vi "PM100D_Plot_ph.vi"(1 "Beam Name":string="Green Unshifted") -> ()   [LabVIEW 2012]
doc: "This VI shows how to communicate with a PM100D optical power/energy meter with SCPI commands.\n- Initializing the instrument\n- Getting system info\n- Setting parameters\n- Measurement configuration\n- Measuring queue\n- Fetching and displaying a measurement value\n- Closing the application"
panel:
  in  "Publish As Adam Channel":bool
  out "Wavelength nm":string="488"
  out "Waveform Chart":dbl(graph)
  out "Readout value":dbl format="%^#_9e"
  out "IDN String":string
  out "Sensor SN":string
  out "Sensor Name":string
  out "Sensor Flags":bool[](array[boolean])
  out "New":bool
  in  "Timeout [ms]":i32=1000
  in  "stop":bool
  in  "Readout Config":string(combo)="POW"
  out "Readout string":string
  out "Error log":string
  in  "Averaging Rate":i32=300
  # "1 Power Sensor"
  # "2 Energy Sensor"
  # "4"
  # "8"
  # "16 Response settable"
  # "32 Wavelength settable"
  # "64 Tau (time constant) settable"
  # "128"
  # "256 With temperature sensor"
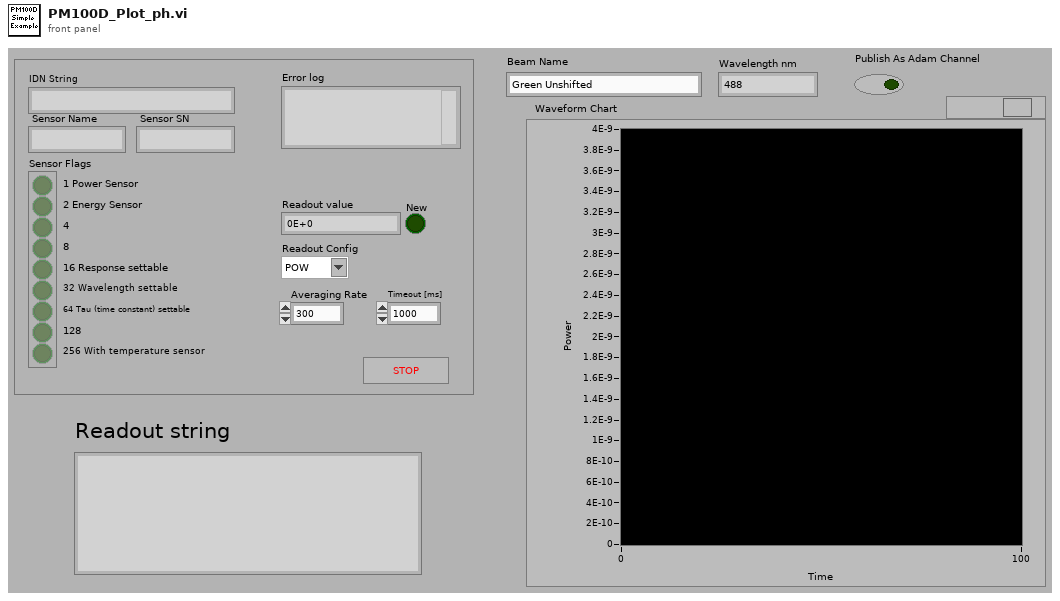
[diagram p1: front panel]
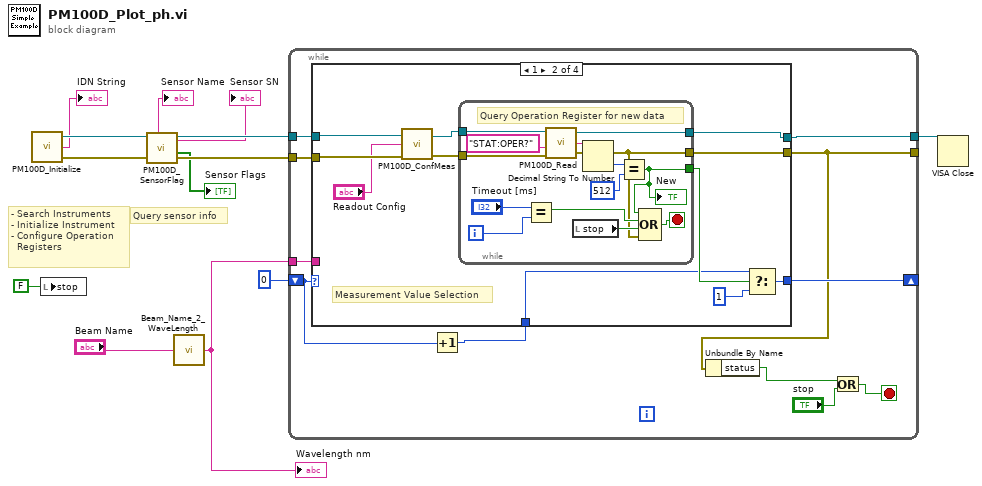
[diagram p0: block diagram]
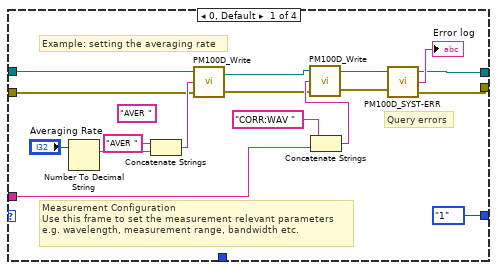
[diagram p2: hidden frame]
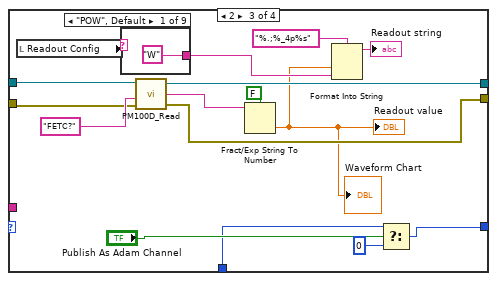
[diagram p3: hidden frame]
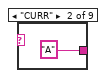
[diagram p4: hidden frame]
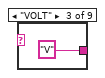
[diagram p5: hidden frame]
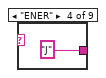
[diagram p6: hidden frame]
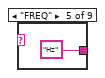
[diagram p7: hidden frame]
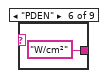
[diagram p8: hidden frame]
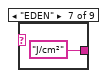
[diagram p9: hidden frame]
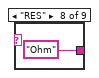
[diagram p10: hidden frame]
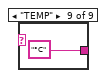
[diagram p11: hidden frame]
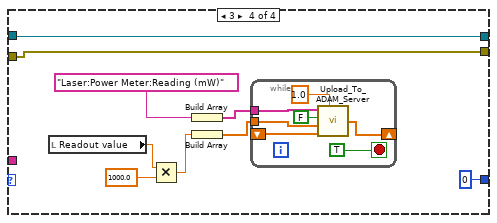
[diagram p12: hidden frame]
diagram:
  # "- Search Instruments\n- Initialize Instrument\n- Configure Operation\n  Registers"
  # "Query sensor info"
  n1 = call "PM100D_Initialize.vi"() -> ("error out"=w12:errorcluster, "Instrument"=→"IDN String":string, "VISA out"=w13:refnum<visa-resource-name>)  [unwired: 3 out]
  n2 = local write "stop"(FALSE ("stop")) -> ()
  n3 = call "PM100D_SensorFlag.vi"("error in (no error)"=w12, "VISA in"=w13) -> ("error out"=w10:errorcluster, "flags"=→"Sensor Flags":bool[], "VISA out"=w11:refnum<visa-resource-name>, "sn"=→"Sensor SN":string, "name"=→"Sensor Name":string)  [unwired: 5 out]
  n4 = call "Beam_Name_2_WaveLength.vi"("Beam Name"="Beam Name") -> ("Wavelength nm"=w3:string)
  "Wavelength nm" <- w3
  n5 = while {
    tunnel: w11 -> [w24]
    tunnel: w10 -> [w23]
    shift-right: [w22] -> _
    shift-left: 0 -> [w19]
    tunnel: [w21] -> w1
    tunnel: [w15] -> _
    tunnel: w3 -> [w20]
    stop <- w16 stop-if-true
    n6 = Increment(x=w19) -> (x+1=w18:i32)
    n7 = case shown="1" w19 {
      tunnel: w24 -> [w38 w52 w81 w100]
      tunnel: w23 -> [w35 w51 w80 w99]
      tunnel: [enum16{"0", "1", "2"}."1" w46 w69 0 ("f")] -> w22
      tunnel: [w33 w48 w79 w100] -> w21
      tunnel: [w32 w47 w72 w99] -> w15
      tunnel: w20 -> [w29 _ _ _]
      tunnel: w18 -> [_ w43 w68 _]
      frame 0, Default {
        (unwired) "AVER " ("string")
        # "Query errors"
        # "Example: setting the averaging rate"
        # "Measurement Configuration\nUse this frame to set the measurement relevant parameters\ne.g. wavelength, measurement range, bandwidth etc."
        n8 = Number To Decimal String(number="Averaging Rate") -> (decimal integer string=w40:string)  [unwired: 1 out]
        n9 = Concatenate Strings("AVER " ("string"), w40) -> (w37:string)
        n10 = call "PM100D_Write.vi"("error in (no error)"=w35, "Command"=w37, "VISA in"=w38) -> ("error out"=w27:errorcluster, "VISA out"=w28:refnum<visa-resource-name>)
        n11 = Concatenate Strings("CORR:WAV " ("string"), w29) -> (w31:string)
        n12 = call "PM100D_Write.vi"("error in (no error)"=w27, "Command"=w31, "VISA in"=w28) -> ("error out"=w26:errorcluster, "VISA out"=w25:refnum<visa-resource-name>)
        n13 = call "PM100D_SYST-ERR.vi"("error out 2"=w26, "VISA In"=w25) -> ("error out"=w32:errorcluster, "Error"=→"Error log":string, "VISA Out"=w33:refnum<visa-resource-name>)  [unwired: 1 out]
      }
      frame 1 {
        # "Measurement Value Selection"
        n14 = call "PM100D_ConfMeas.vi"("error in"=w51, "Conf:"="Readout Config", "VISA In"=w52) -> ("error out"=w49:errorcluster, "dup VISA session"=w50:refnum<visa-resource-name>)
        n15 = while {
          tunnel: w50 -> [w62]
          tunnel: w49 -> [w61]
          tunnel: [w60] -> w48
          tunnel: [w53] -> w47
          tunnel: [w54] -> w45
          i -> [w56]
          stop <- w58 stop-if-true
          # "Query Operation Register for new data"
          n16 = Equal?(x="Timeout [ms]", y=w56) -> (x = y?=w55:bool)
          n17 = call "PM100D_Read.vi"("error in (no error)"=w61, "Command"="STAT:OPER?", "VISA in"=w62) -> ("error out"=w53:errorcluster, "ReadValue"=w65:string, "VISA out"=w60:refnum<visa-resource-name>)  [unwired: 1 out]
          n18 = local read "stop"() -> (w59:bool)
          n19 = Decimal String To Number(string=w65) -> (number=w64:i32)  [unwired: 2 in, 1 out]
          n20 = Equal?(x=w64, y=512) -> (x = y?=w54:bool)
          "New" <- w54
          n21 = Compound Arithmetic op=OR(w54, w55, w59, w53) -> (w58:bool)
        }
        n22 = Select(t=w43, s=w45, f=1) -> (s? t:f=w46:i32)
      }
      frame 2 {
        n23 = local read "Readout Config"() -> (w78:string)
        n24 = case shown="\"POW\", Default" w78 {
          tunnel: ["W" "A" "V" "J" "Hz" "W/cm²" "J/cm²" "Ohm" "°C"] -> w74
          frame "POW", Default {
          }
          frame "CURR" {
          }
          frame "VOLT" {
          }
          frame "ENER" {
          }
          frame "FREQ" {
          }
          frame "PDEN" {
          }
          frame "EDEN" {
          }
          frame "RES" {
          }
          frame "TEMP" {
          }
        }
        n25 = call "PM100D_Read.vi"("error in (no error)"=w80, "Command"="FETC?", "VISA in"=w81) -> ("error out"=w72:errorcluster, "ReadValue"=w77:string, "VISA out"=w79:refnum<visa-resource-name>)  [unwired: 1 out]
        n26 = Fract/Exp String To Number(use system decimal point (T)=FALSE, string=w77) -> (number=w71:dbl)  [unwired: 3 out]
        "Readout value" <- w71
        "Waveform Chart" <- w71
        n27 = Format Into String(format string="%.;%_4p%s", w71, w74) -> (resulting string=→"Readout string":string)  [unwired: 2 in, 1 out]
        n28 = Select(t=w68, s="Publish As Adam Channel", f=0) -> (s? t:f=w69:i32)
      }
      frame 3 {
        n29 = local read "Readout value"() -> (w94:dbl)
        n30 = Multiply(x=w94, y=1000.0) -> (x*y=w92:dbl)
        n31 = Build Array("Laser:Power Meter:Reading (mW)" ("String")) -> (w95:string[])
        n32 = Build Array(w92) -> (w96:dbl[])
        n33 = while {
          shift-right: [w107] -> _
          shift-left: _ -> [w106]
          tunnel: w96 -> [w103]
          tunnel: w95 -> [w102]
          stop <- TRUE stop-if-true
          n34 = call "Upload_To_ADAM_Server.vi"("Averaging Period (s)"=1.0, "Shift In"=w106, "Channel Values"=w103, "Give Variance"=FALSE, "Channel Names"=w102) -> ("Shift Out"=w107:dbl[])  [unwired: 1 in]
        }
      }
    }
    n35 = Unbundle By Name(w15) -> ("status"=w14:bool)
    n36 = Or(x=w14, y="stop") -> (x .or. y?=w16:bool)
  }
  n37 = VISA Close(VISA resource name=w1) -> ()  [unwired: 1 in, 1 out]
